vi "Limit.vi"(6 "Input":dbl, 8 "Lower sensor sense":enum16{"Active Low", "Active High"}(ring), 9 "Lower DigitalInputDevRef":T1={"DevStatus"={"status"=FALSE, "code"=0, "source"=""}, "DIO Channel"=enum."Invalid", "Digital Module"=enum."Digital Module 1"}, 10 "Upper sensor sense":enum16{"Active Low", "Active High"}(ring), 11 "Upper DigitalInputDevRef":T1={"DevStatus"={"status"=FALSE, "code"=0, "source"=""}, "DIO Channel"=enum."Invalid", "Digital Module"=enum."Digital Module 1"}) -> (3 "Output":dbl)   [LabVIEW 2013]
uses:
  <vilib>/Rock Robotics/WPI/DigitalInput/WPI_DigitalInputDevRef.ctl
  <vilib>/Rock Robotics/SystemInterfaces/DIO/FPGA_DIOChannel.ctl
  <vilib>/Rock Robotics/SystemInterfaces/Typedef/FPGA_TypedefDigitalModule.ctl
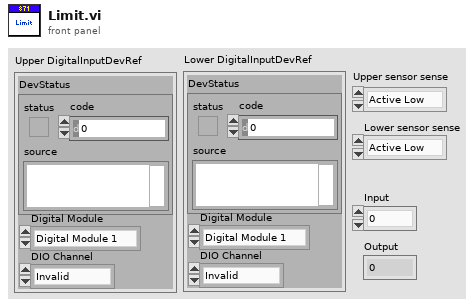
[diagram p1: front panel]
types:
  T1 = typedef "WPI_DigitalInputDevRef.ctl" = cluster{"DevStatus":errorcluster, "DIO Channel":T2, "Digital Module":T3}
  T2 = typedef "FPGA_DIOChannel.ctl" = enum8{"DIO 1", "DIO 2", "DIO 3", "DIO 4", "DIO 5", "DIO 6", "DIO 7", "DIO 8", "DIO 9", "DIO 10", "DIO 11", "DIO 12", "DIO 13", "DIO 14", "Invalid"}
  T3 = typedef "FPGA_TypedefDigitalModule.ctl" = enum16{"Digital Module 1", "Digital Module 2"}
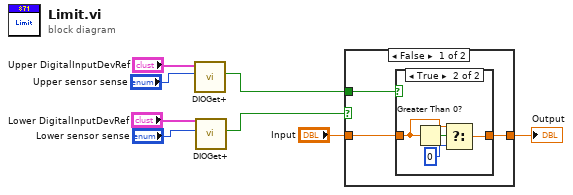
[diagram p0: block diagram]
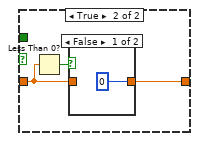
[diagram p3: hidden frame]
diagram:
  n1 = call "DIOGet+.vi"("Sensor Type"="Upper sensor sense", "DigitalInputDevRefIn"="Upper DigitalInputDevRef") -> ("Value"=w3:bool)  [unwired: 7 in, 2 out]
  n2 = call "DIOGet+.vi"("Sensor Type"="Lower sensor sense", "DigitalInputDevRefIn"="Lower DigitalInputDevRef") -> ("Value"=w4:bool)  [unwired: 7 in, 2 out]
  n3 = case shown="False" w4 {
    tunnel: [w9 w19] -> w1
    tunnel: "Input" -> [w10 w18]
    tunnel: w3 -> [w11 _]
    frame False {
      n4 = case shown="True" w11 {
        tunnel: w10 -> [w12 w13]
        tunnel: [w12 w15] -> w9
        frame False {
        }
        frame True {
          n5 = Greater Than 0?(x=w13) -> (x > 0?=w14:bool)
          n6 = Select(t=w13, s=w14, f=0) -> (s? t:f=w15:dbl)
        }
      }
    }
    frame True {
      n7 = Less Than 0?(x=w18) -> (x < 0?=w17:bool)
      n8 = case shown="False" w17 {
        tunnel: [0 w21] -> w19
        tunnel: w18 -> [_ w21]
        frame False {
        }
        frame True {
        }
      }
    }
  }
  "Output" <- w1
